vi "BRig_RT__Case_Exp__State_initTrial__LC_Cue__v3.vi"(6 "input_arrTrig":bool[](array[boolean]), 8 "input_dataTrial":u16[][](array[numeric]), 9 "input_dataExp":u16[](array[numeric]), 10 "input_dataLC":u16[](array[numeric]), 11 "input_dataCurrent":u16[](array[numeric])) -> (0 "output_dataTrial":u16[][](array[numeric]), 3 "output_dataCurrent":u16[](array[numeric]), 4 "output_arrTrig":bool[](array[boolean]))   [LabVIEW 2014]
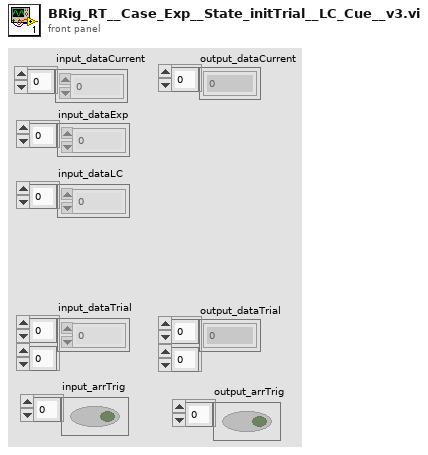
[diagram p1: front panel]
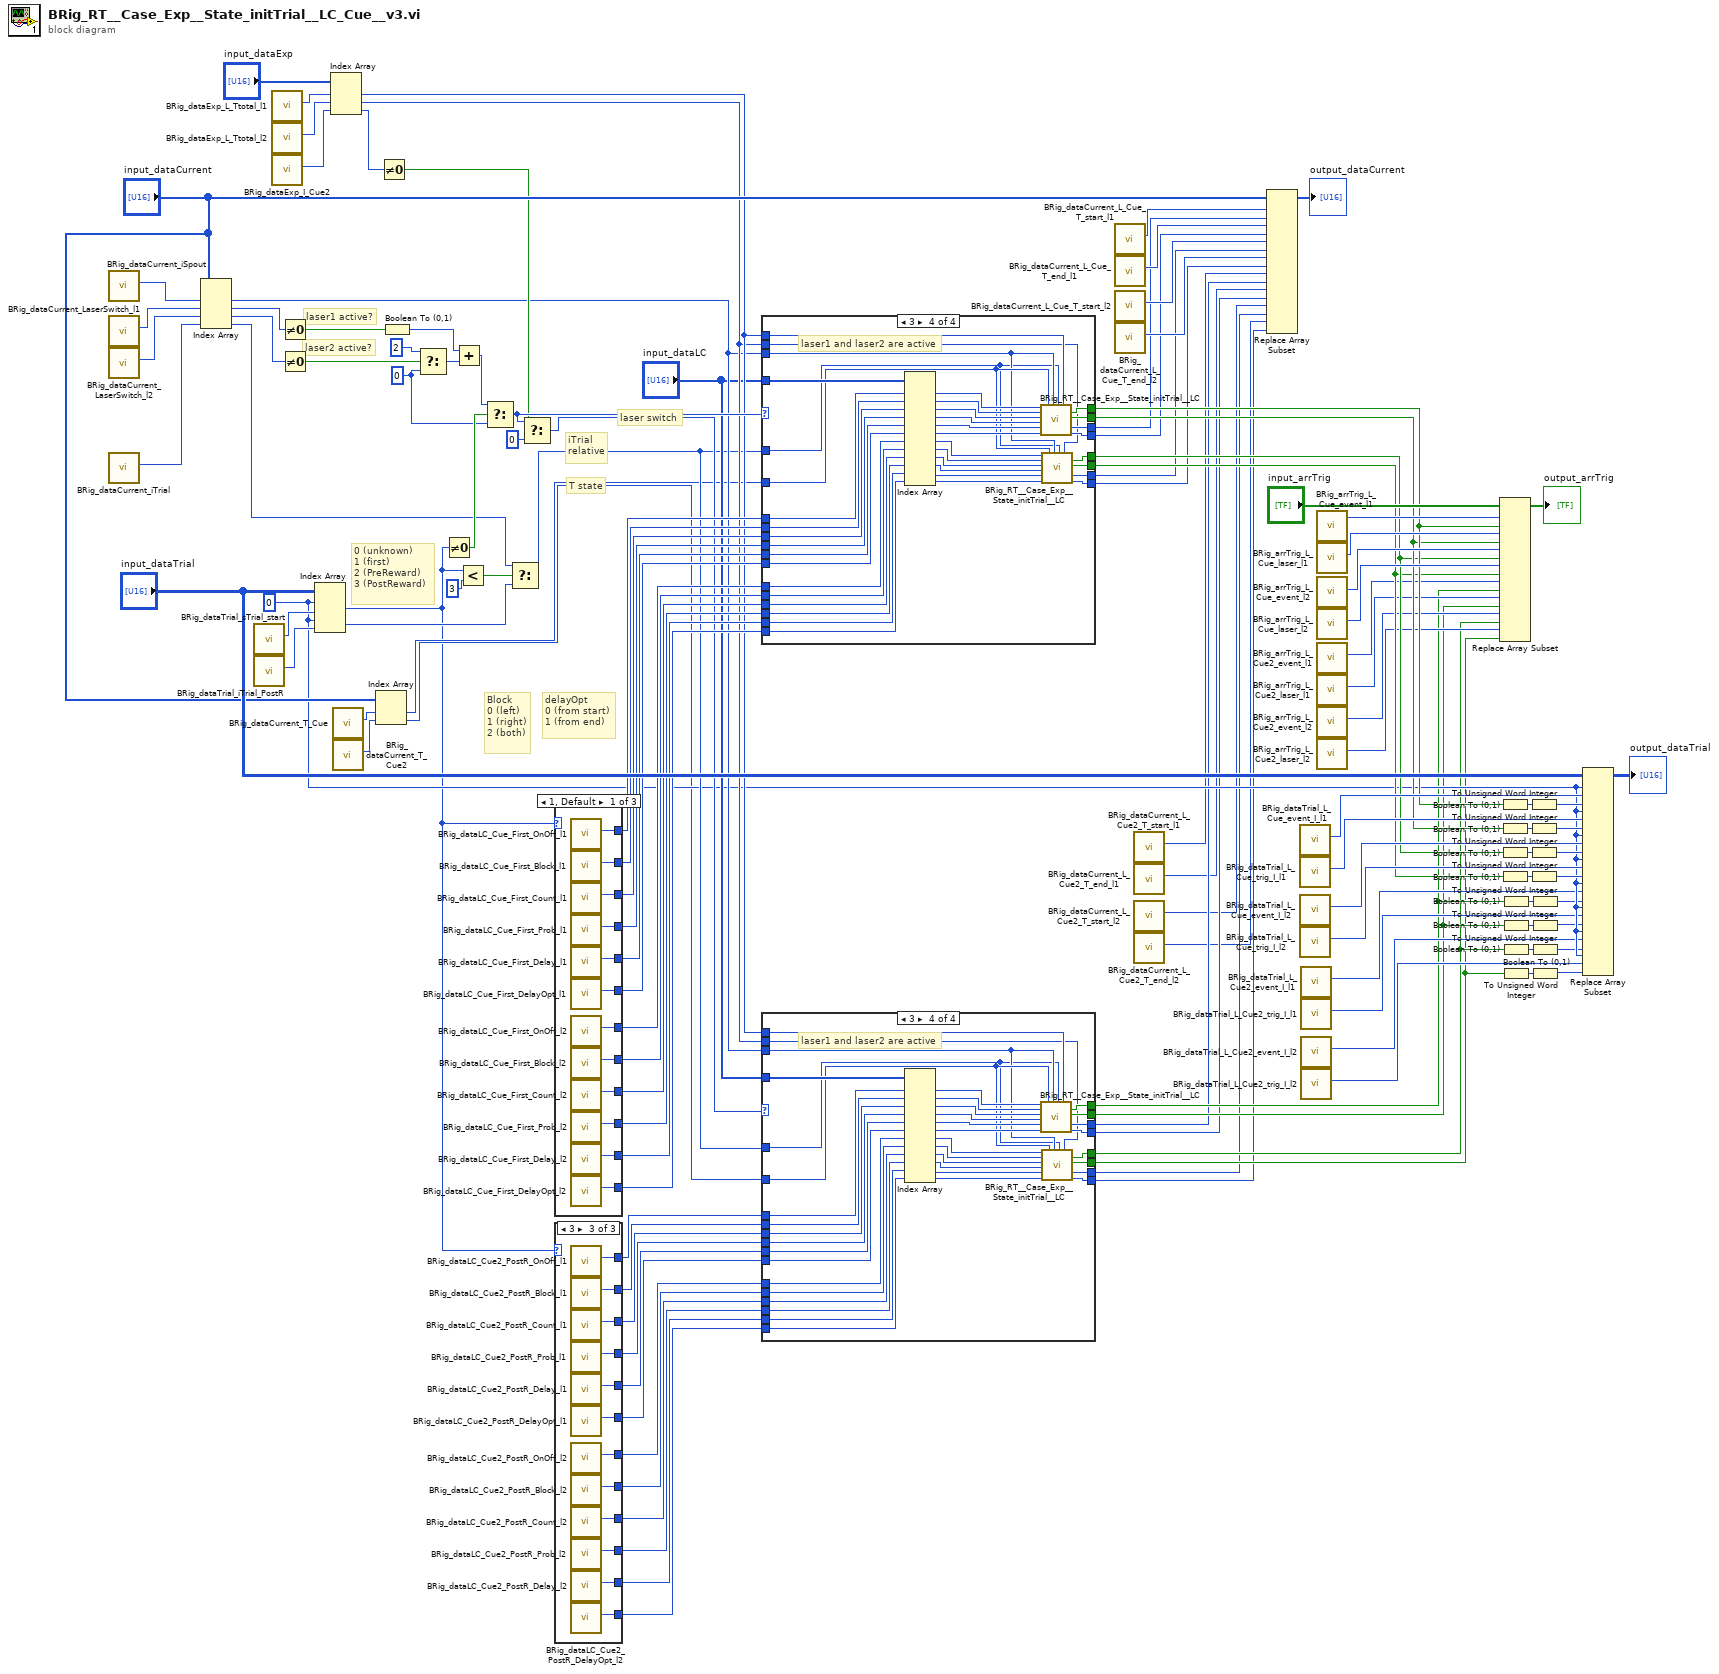
[diagram p0: block diagram]
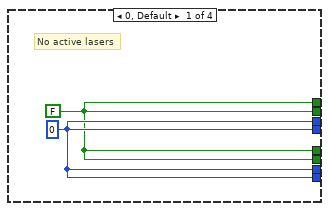
[diagram p2: hidden frame]
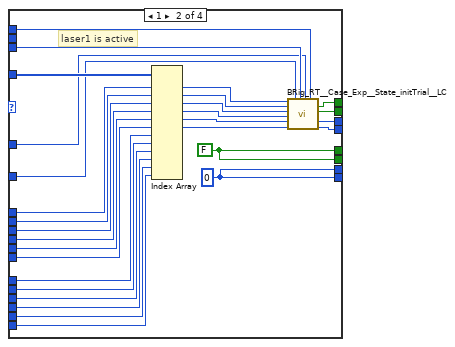
[diagram p3: hidden frame]
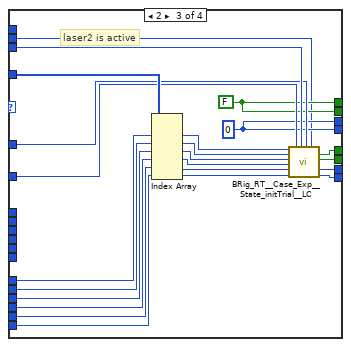
[diagram p4: hidden frame]
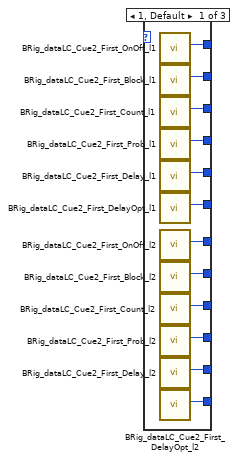
[diagram p5: hidden frame]
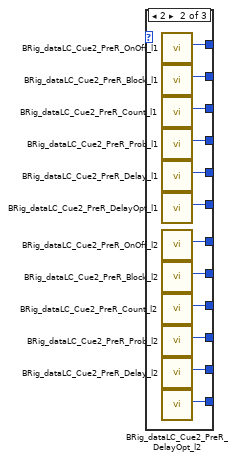
[diagram p6: hidden frame]
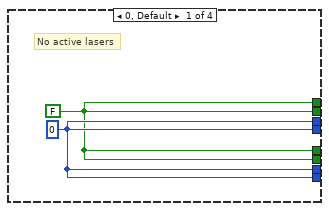
[diagram p7: hidden frame]
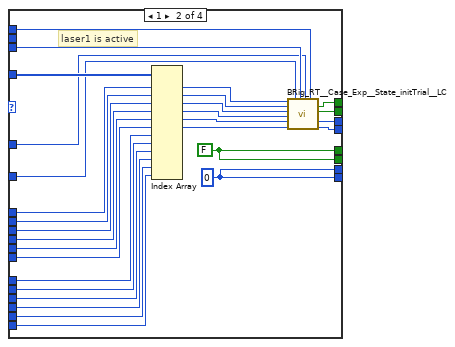
[diagram p8: hidden frame]
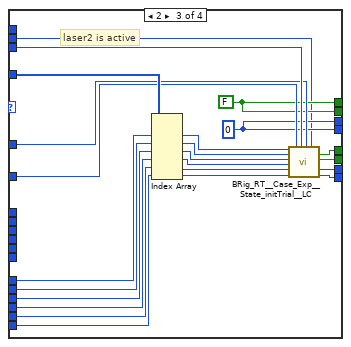
[diagram p9: hidden frame]
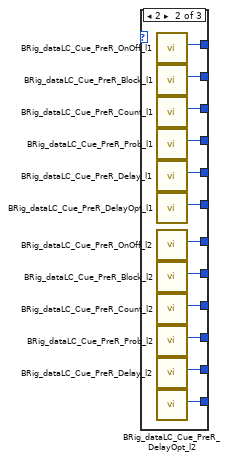
[diagram p10: hidden frame]
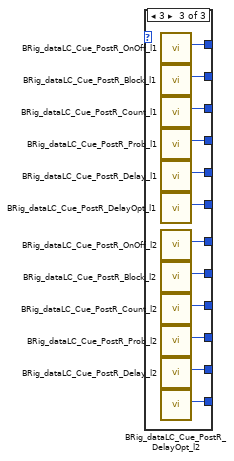
[diagram p11: hidden frame]
diagram:
  w25 = 0
  w115 = i16 0 ("f")
  # "iTrial\nrelative"
  # "laser switch"
  # "T state"
  # "delayOpt\n0 (from start)\n1 (from end)"
  # "Block\n0 (left)\n1 (right)\n2 (both)"
  # "0 (unknown)\n1 (first)\n2 (PreReward)\n3 (PostReward)"
  # "laser2 active?"
  # "laser1 active?"
  n1 = call "BRig_dataCurrent_iSpout.vi"() -> ("output_iSpout"=w113:i32)  [unwired: 11 in]
  n2 = call "BRig_dataCurrent_LaserSwitch_l1.vi"() -> ("output_LaserSwitch_l1"=w126:i32)  [unwired: 11 in]
  n3 = call "BRig_dataCurrent_LaserSwitch_l2.vi"() -> ("output_LaserSwitch_l2"=w125:i32)  [unwired: 11 in]
  n4 = call "BRig_dataCurrent_iTrial.vi"() -> ("output_iTrial"=w78:i32)  [unwired: 11 in]
  n5 = Index Array(array="input_dataCurrent", index #1=w113, index #2=w126, index #3=w125, index #4=w78) -> (element #1=w49:u16, element #2=w124:u16, element #3=w123:u16, element #4=w77:u16)
  n6 = call "BRig_dataTrial_sTrial_start.vi"() -> ("output_sTrial_start"=w122:i32)  [unwired: 11 in]
  n7 = call "BRig_dataTrial_iTrial_PostR.vi"() -> ("output_iTrial_PostR"=w81:i32)  [unwired: 11 in]
  n8 = call "BRig_dataExp_L_Ttotal_l1.vi"() -> ("output_L_Ttotal_l1"=w83:i32)  [unwired: 11 in]
  n9 = call "BRig_dataExp_L_Ttotal_l2.vi"() -> ("output_L_Ttotal_l2"=w84:i32)  [unwired: 11 in]
  n10 = call "BRig_dataExp_I_Cue2.vi"() -> ("output_I_Cue2"=w56:i32)  [unwired: 11 in]
  n11 = Not Equal To 0?(x=w124) -> (x != 0?=w121:bool)
  n12 = Not Equal To 0?(x=w123) -> (x != 0?=w120:bool)
  n13 = Index Array(array="input_dataTrial", index (row) #1=w25, index (col) #1=w122, index (row) #2=w25, index (col) #2=w81) -> (element #1=w1:u16, element #2=w79:u16)
  n14 = Index Array(array="input_dataExp", index #1=w83, index #2=w84, index #3=w56) -> (element #1=w51:u16, element #2=w50:u16, element #3=w55:u16)
  n15 = call "BRig_dataCurrent_T_Cue.vi"() -> ("output_T_Cue"=w86:i32)  [unwired: 11 in]
  n16 = call "BRig_dataCurrent_T_Cue2.vi"() -> ("output_T_Cue2"=w12:i32)  [unwired: 11 in]
  n17 = Index Array(array="input_dataCurrent", index #1=w86, index #2=w12) -> (element #1=w11:u16, element #2=w10:u16)
  n18 = Not Equal To 0?(x=w55) -> (x != 0?=w52:bool)
  n19 = Boolean To (0,1)(Boolean=w121) -> (0, 1=w117:i16)
  n20 = Select(t=i16 2, s=w120, f=w115) -> (s? t:f=w118:i16)
  n21 = Not Equal To 0?(x=w1) -> (x != 0?=w116:bool)
  n22 = Add(x=w117, y=w118) -> (x+y=w114:i16)
  n23 = Less?(x=w1, y=u16 3) -> (x < y?=w80:bool)
  n24 = Select(t=w114, s=w116, f=w115) -> (s? t:f=w53:i16)
  n25 = Select(t=w77, s=w80, f=w79) -> (s? t:f=w46:u16)
  n26 = Select(t=w53, s=w52, f=i16 0) -> (s? t:f=w47:i16)
  n27 = case shown="1, Default" w1 {
    tunnel: [w127 w150 w161] -> w68
    tunnel: [w128 w139 w160] -> w67
    tunnel: [w129 w140 w159] -> w66
    tunnel: [w130 w141 w158] -> w65
    tunnel: [w131 w142 w157] -> w64
    tunnel: [w132 w143 w156] -> w63
    tunnel: [w133 w149 w155] -> w62
    tunnel: [w134 w144 w154] -> w61
    tunnel: [w135 w145 w153] -> w60
    tunnel: [w136 w146 w152] -> w59
    tunnel: [w137 w147 w151] -> w58
    tunnel: [w138 w148 w162] -> w57
    frame 1, Default {
      n28 = call "BRig_dataLC_Cue_First_OnOff_l1.vi"() -> ("output_Cue_First_OnOff"=w127:i32)  [unwired: 11 in]
      n29 = call "BRig_dataLC_Cue_First_Block_l1.vi"() -> ("output_Cue_First_Block"=w128:i32)  [unwired: 11 in]
      n30 = call "BRig_dataLC_Cue_First_Count_l1.vi"() -> ("output_Cue_First_Count"=w129:i32)  [unwired: 11 in]
      n31 = call "BRig_dataLC_Cue_First_Prob_l1.vi"() -> ("output_Cue_First_Prob"=w130:i32)  [unwired: 11 in]
      n32 = call "BRig_dataLC_Cue_First_Delay_l1.vi"() -> ("output_Cue_First_Delay"=w131:i32)  [unwired: 11 in]
      n33 = call "BRig_dataLC_Cue_First_DelayOpt_l1.vi"() -> ("output_Cue_First_DelayOpt"=w132:i32)  [unwired: 11 in]
      n34 = call "BRig_dataLC_Cue_First_OnOff_l2.vi"() -> ("output_Cue_First_OnOff_l2"=w133:i32)  [unwired: 11 in]
      n35 = call "BRig_dataLC_Cue_First_Block_l2.vi"() -> ("output_Cue_First_Block_l2"=w134:i32)  [unwired: 11 in]
      n36 = call "BRig_dataLC_Cue_First_Count_l2.vi"() -> ("output_Cue_First_Count_l2"=w135:i32)  [unwired: 11 in]
      n37 = call "BRig_dataLC_Cue_First_Prob_l2.vi"() -> ("output_Cue_First_Prob_l2"=w136:i32)  [unwired: 11 in]
      n38 = call "BRig_dataLC_Cue_First_Delay_l2.vi"() -> ("output_Cue_First_Delay_l2"=w137:i32)  [unwired: 11 in]
      n39 = call "BRig_dataLC_Cue_First_DelayOpt_l2.vi"() -> ("output_Cue_First_DelayOpt_l2"=w138:i32)  [unwired: 11 in]
    }
    frame 2 {
      n40 = call "BRig_dataLC_Cue_PreR_OnOff_l1.vi"() -> ("output_Cue_PreR_OnOff"=w150:i32)  [unwired: 11 in]
      n41 = call "BRig_dataLC_Cue_PreR_Block_l1.vi"() -> ("output_Cue_PreR_Block"=w139:i32)  [unwired: 11 in]
      n42 = call "BRig_dataLC_Cue_PreR_Count_l1.vi"() -> ("output_Cue_PreR_Count"=w140:i32)  [unwired: 11 in]
      n43 = call "BRig_dataLC_Cue_PreR_Prob_l1.vi"() -> ("output_Cue_PreR_Prob"=w141:i32)  [unwired: 11 in]
      n44 = call "BRig_dataLC_Cue_PreR_Delay_l1.vi"() -> ("output_Cue_PreR_Delay"=w142:i32)  [unwired: 11 in]
      n45 = call "BRig_dataLC_Cue_PreR_DelayOpt_l1.vi"() -> ("output_Cue_PreR_DelayOpt"=w143:i32)  [unwired: 11 in]
      n46 = call "BRig_dataLC_Cue_PreR_OnOff_l2.vi"() -> ("output_Cue_PreR_OnOff_l2"=w149:i32)  [unwired: 11 in]
      n47 = call "BRig_dataLC_Cue_PreR_Block_l2.vi"() -> ("output_Cue_PreR_Block_l2"=w144:i32)  [unwired: 11 in]
      n48 = call "BRig_dataLC_Cue_PreR_Count_l2.vi"() -> ("output_Cue_PreR_Count_l2"=w145:i32)  [unwired: 11 in]
      n49 = call "BRig_dataLC_Cue_PreR_Prob_l2.vi"() -> ("output_Cue_PreR_Prob_l2"=w146:i32)  [unwired: 11 in]
      n50 = call "BRig_dataLC_Cue_PreR_Delay_l2.vi"() -> ("output_Cue_PreR_Delay_l2"=w147:i32)  [unwired: 11 in]
      n51 = call "BRig_dataLC_Cue_PreR_DelayOpt_l2.vi"() -> ("output_Cue_PreR_DelayOpt_l2"=w148:i32)  [unwired: 11 in]
    }
    frame 3 {
      n52 = call "BRig_dataLC_Cue_PostR_OnOff_l1.vi"() -> ("output_Cue_PostR_OnOff"=w161:i32)  [unwired: 11 in]
      n53 = call "BRig_dataLC_Cue_PostR_Block_l1.vi"() -> ("output_Cue_PostR_Block"=w160:i32)  [unwired: 11 in]
      n54 = call "BRig_dataLC_Cue_PostR_Count_l1.vi"() -> ("output_Cue_PostR_Count"=w159:i32)  [unwired: 11 in]
      n55 = call "BRig_dataLC_Cue_PostR_Prob_l1.vi"() -> ("output_Cue_PostR_Prob"=w158:i32)  [unwired: 11 in]
      n56 = call "BRig_dataLC_Cue_PostR_Delay_l1.vi"() -> ("output_Cue_PostR_Delay"=w157:i32)  [unwired: 11 in]
      n57 = call "BRig_dataLC_Cue_PostR_DelayOpt_l1.vi"() -> ("output_Cue_PostR_DelayOpt"=w156:i32)  [unwired: 11 in]
      n58 = call "BRig_dataLC_Cue_PostR_OnOff_l2.vi"() -> ("output_Cue_PostR_OnOff_l2"=w155:i32)  [unwired: 11 in]
      n59 = call "BRig_dataLC_Cue_PostR_Block_l2.vi"() -> ("output_Cue_PostR_Block_l2"=w154:i32)  [unwired: 11 in]
      n60 = call "BRig_dataLC_Cue_PostR_Count_l2.vi"() -> ("output_Cue_PostR_Count_l2"=w153:i32)  [unwired: 11 in]
      n61 = call "BRig_dataLC_Cue_PostR_Prob_l2.vi"() -> ("output_Cue_PostR_Prob_l2"=w152:i32)  [unwired: 11 in]
      n62 = call "BRig_dataLC_Cue_PostR_Delay_l2.vi"() -> ("output_Cue_PostR_Delay_l2"=w151:i32)  [unwired: 11 in]
      n63 = call "BRig_dataLC_Cue_PostR_DelayOpt_l2.vi"() -> ("output_Cue_PostR_DelayOpt_l2"=w162:i32)  [unwired: 11 in]
    }
  }
  n64 = case shown="3" w1 {
    tunnel: [w174 w186 w198] -> w45
    tunnel: [w173 w185 w197] -> w44
    tunnel: [w172 w184 w196] -> w43
    tunnel: [w171 w183 w195] -> w42
    tunnel: [w170 w182 w194] -> w41
    tunnel: [w169 w181 w193] -> w40
    tunnel: [w168 w180 w192] -> w39
    tunnel: [w167 w179 w191] -> w38
    tunnel: [w166 w178 w190] -> w37
    tunnel: [w165 w177 w189] -> w36
    tunnel: [w164 w176 w188] -> w35
    tunnel: [w163 w175 w187] -> w34
    frame 1, Default {
      n65 = call "BRig_dataLC_Cue2_First_OnOff_l1.vi"() -> ("output_Cue2_First_OnOff"=w174:i32)  [unwired: 11 in]
      n66 = call "BRig_dataLC_Cue2_First_Block_l1.vi"() -> ("output_Cue2_First_Block"=w173:i32)  [unwired: 11 in]
      n67 = call "BRig_dataLC_Cue2_First_Count_l1.vi"() -> ("output_Cue2_First_Count"=w172:i32)  [unwired: 11 in]
      n68 = call "BRig_dataLC_Cue2_First_Prob_l1.vi"() -> ("output_Cue2_First_Prob"=w171:i32)  [unwired: 11 in]
      n69 = call "BRig_dataLC_Cue2_First_Delay_l1.vi"() -> ("output_Cue2_First_Delay"=w170:i32)  [unwired: 11 in]
      n70 = call "BRig_dataLC_Cue2_First_DelayOpt_l1.vi"() -> ("output_Cue2_First_DelayOpt"=w169:i32)  [unwired: 11 in]
      n71 = call "BRig_dataLC_Cue2_First_OnOff_l2.vi"() -> ("output_Cue2_First_OnOff_l2"=w168:i32)  [unwired: 11 in]
      n72 = call "BRig_dataLC_Cue2_First_Block_l2.vi"() -> ("output_Cue2_First_Block_l2"=w167:i32)  [unwired: 11 in]
      n73 = call "BRig_dataLC_Cue2_First_Count_l2.vi"() -> ("output_Cue2_First_Count_l2"=w166:i32)  [unwired: 11 in]
      n74 = call "BRig_dataLC_Cue2_First_Prob_l2.vi"() -> ("output_Cue2_First_Prob_l2"=w165:i32)  [unwired: 11 in]
      n75 = call "BRig_dataLC_Cue2_First_Delay_l2.vi"() -> ("output_Cue2_First_Delay_l2"=w164:i32)  [unwired: 11 in]
      n76 = call "BRig_dataLC_Cue2_First_DelayOpt_l2.vi"() -> ("output_Cue2_First_DelayOpt_l2"=w163:i32)  [unwired: 11 in]
    }
    frame 2 {
      n77 = call "BRig_dataLC_Cue2_PreR_OnOff_l1.vi"() -> ("output_Cue2_PreR_OnOff"=w186:i32)  [unwired: 11 in]
      n78 = call "BRig_dataLC_Cue2_PreR_Block_l1.vi"() -> ("output_Cue2_PreR_Block"=w185:i32)  [unwired: 11 in]
      n79 = call "BRig_dataLC_Cue2_PreR_Count_l1.vi"() -> ("output_Cue2_PreR_Count"=w184:i32)  [unwired: 11 in]
      n80 = call "BRig_dataLC_Cue2_PreR_Prob_l1.vi"() -> ("output_Cue2_PreR_Prob"=w183:i32)  [unwired: 11 in]
      n81 = call "BRig_dataLC_Cue2_PreR_Delay_l1.vi"() -> ("output_Cue2_PreR_Delay"=w182:i32)  [unwired: 11 in]
      n82 = call "BRig_dataLC_Cue2_PreR_DelayOpt_l1.vi"() -> ("output_Cue2_PreR_DelayOpt"=w181:i32)  [unwired: 11 in]
      n83 = call "BRig_dataLC_Cue2_PreR_OnOff_l2.vi"() -> ("output_Cue2_PreR_OnOff_l2"=w180:i32)  [unwired: 11 in]
      n84 = call "BRig_dataLC_Cue2_PreR_Block_l2.vi"() -> ("output_Cue2_PreR_Block_l2"=w179:i32)  [unwired: 11 in]
      n85 = call "BRig_dataLC_Cue2_PreR_Count_l2.vi"() -> ("output_Cue2_PreR_Count_l2"=w178:i32)  [unwired: 11 in]
      n86 = call "BRig_dataLC_Cue2_PreR_Prob_l2.vi"() -> ("output_Cue2_PreR_Prob_l2"=w177:i32)  [unwired: 11 in]
      n87 = call "BRig_dataLC_Cue2_PreR_Delay_l2.vi"() -> ("output_Cue2_PreR_Delay_l2"=w176:i32)  [unwired: 11 in]
      n88 = call "BRig_dataLC_Cue2_PreR_DelayOpt_l2.vi"() -> ("output_Cue2_PreR_DelayOpt_l2"=w175:i32)  [unwired: 11 in]
    }
    frame 3 {
      n89 = call "BRig_dataLC_Cue2_PostR_OnOff_l1.vi"() -> ("output_Cue2_PostR_OnOff"=w198:i32)  [unwired: 11 in]
      n90 = call "BRig_dataLC_Cue2_PostR_Block_l1.vi"() -> ("output_Cue2_PostR_Block"=w197:i32)  [unwired: 11 in]
      n91 = call "BRig_dataLC_Cue2_PostR_Count_l1.vi"() -> ("output_Cue2_PostR_Count"=w196:i32)  [unwired: 11 in]
      n92 = call "BRig_dataLC_Cue2_PostR_Prob_l1.vi"() -> ("output_Cue2_PostR_Prob"=w195:i32)  [unwired: 11 in]
      n93 = call "BRig_dataLC_Cue2_PostR_Delay_l1.vi"() -> ("output_Cue2_PostR_Delay"=w194:i32)  [unwired: 11 in]
      n94 = call "BRig_dataLC_Cue2_PostR_DelayOpt_l1.vi"() -> ("output_Cue2_PostR_DelayOpt"=w193:i32)  [unwired: 11 in]
      n95 = call "BRig_dataLC_Cue2_PostR_OnOff_l2.vi"() -> ("output_Cue2_PostR_OnOff_l2"=w192:i32)  [unwired: 11 in]
      n96 = call "BRig_dataLC_Cue2_PostR_Block_l2.vi"() -> ("output_Cue2_PostR_Block_l2"=w191:i32)  [unwired: 11 in]
      n97 = call "BRig_dataLC_Cue2_PostR_Count_l2.vi"() -> ("output_Cue2_PostR_Count_l2"=w190:i32)  [unwired: 11 in]
      n98 = call "BRig_dataLC_Cue2_PostR_Prob_l2.vi"() -> ("output_Cue2_PostR_Prob_l2"=w189:i32)  [unwired: 11 in]
      n99 = call "BRig_dataLC_Cue2_PostR_Delay_l2.vi"() -> ("output_Cue2_PostR_Delay_l2"=w188:i32)  [unwired: 11 in]
      n100 = call "BRig_dataLC_Cue2_PostR_DelayOpt_l2.vi"() -> ("output_Cue2_PostR_DelayOpt_l2"=w187:i32)  [unwired: 11 in]
    }
  }
  n101 = case shown="3" w53 {
    tunnel: "input_dataLC" -> [_ w229 w252 w290]
    tunnel: w49 -> [_ w221 w244 w276]
    tunnel: w11 -> [_ w222 w245 w277]
    tunnel: w46 -> [_ w220 w243 w275]
    tunnel: [w199 w219 w232 w274] -> w76
    tunnel: [w199 w218 w232 w273] -> w75
    tunnel: [w200 w217 w231 w272] -> w74
    tunnel: [w200 w216 w231 w271] -> w73
    tunnel: [w199 w203 w242 w270] -> w71
    tunnel: [w200 w202 w241 w269] -> w70
    tunnel: [w199 w203 w240 w268] -> w72
    tunnel: [w200 w202 w239 w267] -> w69
    tunnel: w68 -> [_ w215 _ w266]
    tunnel: w67 -> [_ w214 _ w265]
    tunnel: w66 -> [_ w213 _ w264]
    tunnel: w65 -> [_ w212 _ w263]
    tunnel: w64 -> [_ w211 _ w262]
    tunnel: w63 -> [_ w210 _ w261]
    tunnel: w62 -> [_ w209 w238 w260]
    tunnel: w61 -> [_ w208 w237 w259]
    tunnel: w60 -> [_ w207 w236 w258]
    tunnel: w59 -> [_ w206 w235 w257]
    tunnel: w58 -> [_ w205 w234 w256]
    tunnel: w57 -> [_ w204 w233 w255]
    tunnel: w51 -> [_ w201 _ w254]
    tunnel: w50 -> [_ _ w230 w253]
    frame 0, Default {
      w200 = u16 0
      w199 = FALSE
      # "No active lasers"
    }
    frame 1 {
      w202 = u16 0
      w203 = FALSE
      # "laser1 is active"
      n102 = Index Array(array=w229, index #1=w215, index #2=w214, index #3=w213, index #4=w212, index #5=w211, index #6=w210, index #7=w209, index #8=w208, index #9=w207, index #10=w206, index #11=w205, index #12=w204) -> (element #1=w228:u16, element #2=w227:u16, element #3=w226:u16, element #4=w225:u16, element #5=w224:u16, element #6=w223:u16)  [unwired: 6 out]
      n103 = call "BRig_RT__Case_Exp__State_initTrial__LC.vi"("input_L_OnOff"=w228, "input_L_Block"=w227, "input_L_Count"=w226, "input_L_Prob"=w225, "input_L_Tdelay"=w224, "input_L_delayOpt"=w223, "input_T_state"=w222, "input_iSpout"=w221, "input_iTrial_relative"=w220, "input_L_T"=w201) -> ("output_LC_Event"=w219:bool, "output_LC_Laser"=w218:bool, "output_L_Tstart"=w217:u16, "output_L_Tend"=w216:u16)  [unwired: 6 in]
    }
    frame 2 {
      w231 = u16 0
      w232 = FALSE
      # "laser2 is active"
      n104 = Index Array(array=w252, index #1=w238, index #2=w237, index #3=w236, index #4=w235, index #5=w234, index #6=w233) -> (element #1=w246:u16, element #2=w247:u16, element #3=w248:u16, element #4=w249:u16, element #5=w250:u16, element #6=w251:u16)
      n105 = call "BRig_RT__Case_Exp__State_initTrial__LC.vi"("input_L_OnOff"=w246, "input_L_Block"=w247, "input_L_Count"=w248, "input_L_Prob"=w249, "input_L_Tdelay"=w250, "input_L_delayOpt"=w251, "input_T_state"=w245, "input_iSpout"=w244, "input_iTrial_relative"=w243, "input_L_T"=w230) -> ("output_LC_Event"=w240:bool, "output_LC_Laser"=w242:bool, "output_L_Tstart"=w241:u16, "output_L_Tend"=w239:u16)  [unwired: 6 in]
    }
    frame 3 {
      # "laser1 and laser2 are active"
      n106 = Index Array(array=w290, index #1=w266, index #2=w265, index #3=w264, index #4=w263, index #5=w262, index #6=w261, index #7=w260, index #8=w259, index #9=w258, index #10=w257, index #11=w256, index #12=w255) -> (element #1=w289:u16, element #2=w288:u16, element #3=w287:u16, element #4=w286:u16, element #5=w285:u16, element #6=w284:u16, element #7=w278:u16, element #8=w279:u16, element #9=w280:u16, element #10=w281:u16, element #11=w282:u16, element #12=w283:u16)
      n107 = call "BRig_RT__Case_Exp__State_initTrial__LC.vi"("input_L_OnOff"=w289, "input_L_Block"=w288, "input_L_Count"=w287, "input_L_Prob"=w286, "input_L_Tdelay"=w285, "input_L_delayOpt"=w284, "input_T_state"=w277, "input_iSpout"=w276, "input_iTrial_relative"=w275, "input_L_T"=w254) -> ("output_LC_Event"=w274:bool, "output_LC_Laser"=w273:bool, "output_L_Tstart"=w272:u16, "output_L_Tend"=w271:u16)  [unwired: 6 in]
      n108 = call "BRig_RT__Case_Exp__State_initTrial__LC.vi"("input_L_OnOff"=w278, "input_L_Block"=w279, "input_L_Count"=w280, "input_L_Prob"=w281, "input_L_Tdelay"=w282, "input_L_delayOpt"=w283, "input_T_state"=w277, "input_iSpout"=w276, "input_iTrial_relative"=w275, "input_L_T"=w253) -> ("output_LC_Event"=w268:bool, "output_LC_Laser"=w270:bool, "output_L_Tstart"=w269:u16, "output_L_Tend"=w267:u16)  [unwired: 6 in]
    }
  }
  n109 = case shown="3" w47 {
    tunnel: "input_dataLC" -> [_ w321 w344 w382]
    tunnel: w49 -> [_ w313 w336 w368]
    tunnel: w10 -> [_ w314 w337 w369]
    tunnel: w46 -> [_ w312 w335 w367]
    tunnel: [w291 w311 w324 w366] -> w16
    tunnel: [w291 w310 w324 w365] -> w15
    tunnel: [w292 w309 w323 w364] -> w8
    tunnel: [w292 w308 w323 w363] -> w6
    tunnel: [w291 w295 w334 w362] -> w13
    tunnel: [w292 w294 w333 w361] -> w4
    tunnel: [w291 w295 w332 w360] -> w14
    tunnel: [w292 w294 w331 w359] -> w2
    tunnel: w45 -> [_ w307 _ w358]
    tunnel: w44 -> [_ w306 _ w357]
    tunnel: w43 -> [_ w305 _ w356]
    tunnel: w42 -> [_ w304 _ w355]
    tunnel: w41 -> [_ w303 _ w354]
    tunnel: w40 -> [_ w302 _ w353]
    tunnel: w39 -> [_ w301 w330 w352]
    tunnel: w38 -> [_ w300 w329 w351]
    tunnel: w37 -> [_ w299 w328 w350]
    tunnel: w36 -> [_ w298 w327 w349]
    tunnel: w35 -> [_ w297 w326 w348]
    tunnel: w34 -> [_ w296 w325 w347]
    tunnel: w51 -> [_ w293 _ w346]
    tunnel: w50 -> [_ _ w322 w345]
    frame 0, Default {
      w292 = u16 0
      w291 = FALSE
      # "No active lasers"
    }
    frame 1 {
      w294 = u16 0
      w295 = FALSE
      # "laser1 is active"
      n110 = Index Array(array=w321, index #1=w307, index #2=w306, index #3=w305, index #4=w304, index #5=w303, index #6=w302, index #7=w301, index #8=w300, index #9=w299, index #10=w298, index #11=w297, index #12=w296) -> (element #1=w320:u16, element #2=w319:u16, element #3=w318:u16, element #4=w317:u16, element #5=w316:u16, element #6=w315:u16)  [unwired: 6 out]
      n111 = call "BRig_RT__Case_Exp__State_initTrial__LC.vi"("input_L_OnOff"=w320, "input_L_Block"=w319, "input_L_Count"=w318, "input_L_Prob"=w317, "input_L_Tdelay"=w316, "input_L_delayOpt"=w315, "input_T_state"=w314, "input_iSpout"=w313, "input_iTrial_relative"=w312, "input_L_T"=w293) -> ("output_LC_Event"=w311:bool, "output_LC_Laser"=w310:bool, "output_L_Tstart"=w309:u16, "output_L_Tend"=w308:u16)  [unwired: 6 in]
    }
    frame 2 {
      w323 = u16 0
      w324 = FALSE
      # "laser2 is active"
      n112 = Index Array(array=w344, index #1=w330, index #2=w329, index #3=w328, index #4=w327, index #5=w326, index #6=w325) -> (element #1=w338:u16, element #2=w339:u16, element #3=w340:u16, element #4=w341:u16, element #5=w342:u16, element #6=w343:u16)
      n113 = call "BRig_RT__Case_Exp__State_initTrial__LC.vi"("input_L_OnOff"=w338, "input_L_Block"=w339, "input_L_Count"=w340, "input_L_Prob"=w341, "input_L_Tdelay"=w342, "input_L_delayOpt"=w343, "input_T_state"=w337, "input_iSpout"=w336, "input_iTrial_relative"=w335, "input_L_T"=w322) -> ("output_LC_Event"=w332:bool, "output_LC_Laser"=w334:bool, "output_L_Tstart"=w333:u16, "output_L_Tend"=w331:u16)  [unwired: 6 in]
    }
    frame 3 {
      # "laser1 and laser2 are active"
      n114 = Index Array(array=w382, index #1=w358, index #2=w357, index #3=w356, index #4=w355, index #5=w354, index #6=w353, index #7=w352, index #8=w351, index #9=w350, index #10=w349, index #11=w348, index #12=w347) -> (element #1=w381:u16, element #2=w380:u16, element #3=w379:u16, element #4=w378:u16, element #5=w377:u16, element #6=w376:u16, element #7=w370:u16, element #8=w371:u16, element #9=w372:u16, element #10=w373:u16, element #11=w374:u16, element #12=w375:u16)
      n115 = call "BRig_RT__Case_Exp__State_initTrial__LC.vi"("input_L_OnOff"=w381, "input_L_Block"=w380, "input_L_Count"=w379, "input_L_Prob"=w378, "input_L_Tdelay"=w377, "input_L_delayOpt"=w376, "input_T_state"=w369, "input_iSpout"=w368, "input_iTrial_relative"=w367, "input_L_T"=w346) -> ("output_LC_Event"=w366:bool, "output_LC_Laser"=w365:bool, "output_L_Tstart"=w364:u16, "output_L_Tend"=w363:u16)  [unwired: 6 in]
      n116 = call "BRig_RT__Case_Exp__State_initTrial__LC.vi"("input_L_OnOff"=w370, "input_L_Block"=w371, "input_L_Count"=w372, "input_L_Prob"=w373, "input_L_Tdelay"=w374, "input_L_delayOpt"=w375, "input_T_state"=w369, "input_iSpout"=w368, "input_iTrial_relative"=w367, "input_L_T"=w345) -> ("output_LC_Event"=w360:bool, "output_LC_Laser"=w362:bool, "output_L_Tstart"=w361:u16, "output_L_Tend"=w359:u16)  [unwired: 6 in]
    }
  }
  n117 = call "BRig_dataCurrent_L_Cue_T_start_l1.vi"() -> ("outputL_Cue_T_start_l1"=w98:i32)  [unwired: 11 in]
  n118 = call "BRig_dataCurrent_L_Cue_T_end_l1.vi"() -> ("output_L_Cue_T_end_l1"=w97:i32)  [unwired: 11 in]
  n119 = call "BRig_dataCurrent_L_Cue_T_start_l2.vi"() -> ("output_L_Cue_T_start_l2"=w96:i32)  [unwired: 11 in]
  n120 = call "BRig_dataCurrent_L_Cue_T_end_l2.vi"() -> ("output_L_Cue_T_end_l2"=w95:i32)  [unwired: 11 in]
  n121 = call "BRig_dataCurrent_L_Cue2_T_start_l1.vi"() -> ("outputL_Cue2_T_start_l1"=w9:i32)  [unwired: 11 in]
  n122 = call "BRig_dataCurrent_L_Cue2_T_end_l1.vi"() -> ("output_L_Cue2_T_end_l1"=w7:i32)  [unwired: 11 in]
  n123 = call "BRig_dataCurrent_L_Cue2_T_start_l2.vi"() -> ("output_L_Cue2_T_start_l2"=w5:i32)  [unwired: 11 in]
  n124 = call "BRig_dataCurrent_L_Cue2_T_end_l2.vi"() -> ("output_L_Cue2_T_end_l2"=w3:i32)  [unwired: 11 in]
  n125 = Replace Array Subset(array="input_dataCurrent", new element #1=w74, index #1=w98, new element #2=w73, index #2=w97, new element #3=w70, index #3=w96, new element #4=w69, index #4=w95, new element #5=w8, index #5=w9, new element #6=w6, index #6=w7, new element #7=w4, index #7=w5, new element #8=w2, index #8=w3) -> (→"output_dataCurrent":u16[])
  n126 = call "BRig_dataTrial_L_Cue_event_I_l1.vi"() -> ("output_L_Cue_event_I_l1"=w87:i32)  [unwired: 11 in]
  n127 = call "BRig_dataTrial_L_Cue_trig_I_l1.vi"() -> ("output_L_Cue_trig_I_l1"=w89:i32)  [unwired: 11 in]
  n128 = call "BRig_dataTrial_L_Cue_event_I_l2.vi"() -> ("output_L_Cue_event_I_l2"=w88:i32)  [unwired: 11 in]
  n129 = call "BRig_dataTrial_L_Cue_trig_I_l2.vi"() -> ("output_L_Cue_trig_I_l2"=w90:i32)  [unwired: 11 in]
  n130 = call "BRig_dataTrial_L_Cue2_event_I_l1.vi"() -> ("output_L_Cue2_event_I_l1"=w24:i32)  [unwired: 11 in]
  n131 = call "BRig_dataTrial_L_Cue2_trig_I_l1.vi"() -> ("output_L_Cue2_trig_I_l1"=w23:i32)  [unwired: 11 in]
  n132 = call "BRig_dataTrial_L_Cue2_event_I_l2.vi"() -> ("output_L_Cue2_event_I_l2"=w22:i32)  [unwired: 11 in]
  n133 = call "BRig_dataTrial_L_Cue2_trig_I_l2.vi"() -> ("output_L_Cue2_trig_I_l2"=w21:i32)  [unwired: 11 in]
  n134 = call "BRig_arrTrig_L_Cue_event_l1.vi"() -> ("output_L_Cue_event_l1"=w91:i32)  [unwired: 11 in]
  n135 = call "BRig_arrTrig_L_Cue_laser_l1.vi"() -> ("output_L_Cue_laser_l1"=w92:i32)  [unwired: 11 in]
  n136 = call "BRig_arrTrig_L_Cue_event_l2.vi"() -> ("output_L_Cue_event_l2"=w94:i32)  [unwired: 11 in]
  n137 = call "BRig_arrTrig_L_Cue_laser_l2.vi"() -> ("output_L_Cue_laser_l2"=w93:i32)  [unwired: 11 in]
  n138 = call "BRig_arrTrig_L_Cue2_event_l1.vi"() -> ("output_L_Cue2_event_l1"=w33:i32)  [unwired: 11 in]
  n139 = call "BRig_arrTrig_L_Cue2_laser_l1.vi"() -> ("output_L_Cue2_laser_l1"=w32:i32)  [unwired: 11 in]
  n140 = call "BRig_arrTrig_L_Cue2_event_l2.vi"() -> ("output_L_Cue2_event_l2"=w31:i32)  [unwired: 11 in]
  n141 = call "BRig_arrTrig_L_Cue2_laser_l2.vi"() -> ("output_L_Cue2_laser_l2"=w30:i32)  [unwired: 11 in]
  n142 = Replace Array Subset(array="input_arrTrig", new element #1=w76, index #1=w91, new element #2=w75, index #2=w92, new element #3=w72, index #3=w94, new element #4=w71, index #4=w93, new element #5=w16, index #5=w33, new element #6=w15, index #6=w32, new element #7=w14, index #7=w31, new element #8=w13, index #8=w30) -> (→"output_arrTrig":bool[])
  n143 = Boolean To (0,1)(Boolean=w76) -> (0, 1=w109:i16)
  n144 = Boolean To (0,1)(Boolean=w75) -> (0, 1=w108:i16)
  n145 = Boolean To (0,1)(Boolean=w72) -> (0, 1=w106:i16)
  n146 = Boolean To (0,1)(Boolean=w71) -> (0, 1=w107:i16)
  n147 = Boolean To (0,1)(Boolean=w16) -> (0, 1=w29:i16)
  n148 = Boolean To (0,1)(Boolean=w15) -> (0, 1=w28:i16)
  n149 = Boolean To (0,1)(Boolean=w14) -> (0, 1=w26:i16)
  n150 = Boolean To (0,1)(Boolean=w13) -> (0, 1=w27:i16)
  n151 = To Unsigned Word Integer(number=w109) -> (unsigned 16bit integer=w104:u16)
  n152 = To Unsigned Word Integer(number=w108) -> (unsigned 16bit integer=w103:u16)
  n153 = To Unsigned Word Integer(number=w106) -> (unsigned 16bit integer=w102:u16)
  n154 = To Unsigned Word Integer(number=w107) -> (unsigned 16bit integer=w101:u16)
  n155 = To Unsigned Word Integer(number=w29) -> (unsigned 16bit integer=w20:u16)
  n156 = To Unsigned Word Integer(number=w28) -> (unsigned 16bit integer=w19:u16)
  n157 = To Unsigned Word Integer(number=w26) -> (unsigned 16bit integer=w18:u16)
  n158 = To Unsigned Word Integer(number=w27) -> (unsigned 16bit integer=w17:u16)
  n159 = Replace Array Subset(array="input_dataTrial", new element #1=w104, index (row) #1=w25, index (col) #1=w87, new element #2=w103, index (row) #2=w25, index (col) #2=w89, new element #3=w102, index (row) #3=w25, index (col) #3=w88, new element #4=w101, index (row) #4=w25, index (col) #4=w90, new element #5=w20, index (row) #5=w25, index (col) #5=w24, new element #6=w19, index (row) #6=w25, index (col) #6=w23, new element #7=w18, index (row) #7=w25, index (col) #7=w22, new element #8=w17, index (row) #8=w25, index (col) #8=w21) -> (→"output_dataTrial":u16[][])
